vi "Begin.vi"(8 "error in":errorcluster) -> (0 "error out":errorcluster)   [LabVIEW 2016]
doc: "Called before other user functions, this VI is expected to open initial I/O refnums, load in file data, and do all program initialization. Notice that the <B>error out</B> terminal is simply used for data flow. Wiring it to other structures or subVIs ensures that this VI runs first."
uses:
  <vilib>/Rock Robotics/WPI/Joystick/WPI_JoystickDeviceEnum.ctl
  <vilib>/Rock Robotics/WPI/ThirdParty/Sensors/navX/_TypeDefs/FRIC_navX_DeviceNumbersTypeDef.ctl
  <vilib>/Rock Robotics/WPI/ThirdParty/CanMotor/TalonSRX/WPI_CANTalonSRX_APIControlMode.ctl
  <vilib>/Rock Robotics/WPI/ThirdParty/CanMotor/TalonSRX/WPI_CANTalonSRX_BrakeOverride.ctl
  <vilib>/Rock Robotics/SystemInterfaces/DIO/FPGA_DIOPWMChannel.ctl
  <vilib>/Rock Robotics/WPI/SafetyOutput/WPI_SafetyOutputConfigMenu.ctl
  <vilib>/Rock Robotics/WPI/DriverStation/WPI_DriverStationRobotMode2.ctl
  <vilib>/Rock Robotics/Network Tables/NT Write String Array.vi
  Robot Global Data.vi
  <vilib>/Rock Robotics/WPI/Camera/WPI_CameraFrameRate.ctl
  <vilib>/Rock Robotics/WPI/Camera/WPI_CameraImageSize.ctl
  <vilib>/Rock Robotics/WPI/Camera/WPI_CameraWhite Balance Values.ctl
  <vilib>/Rock Robotics/WPI/Camera/WPI_CameraExposure Values.ctl
  <vilib>/Rock Robotics/WPI/RobotDrive/WPI_RobotDriveOpen2MotorWithTalon.vi
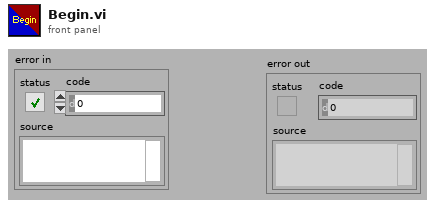
[diagram p1: front panel]
types:
  T1 = typedef "WPI_DriverStationRobotMode2.ctl" = enum16{"Autonomous Disabled", "Autonomous Enabled", "Teleop Disabled", "Teleop Enabled", "Disconnected", "Finish", "Test Disabled", "Test Enabled", "Emergency Stopped"}
  T2 = typedef "WPI_SafetyOutputConfigMenu.ctl" = enum16{"Enable", "Disable"}
  T3 = typedef "FPGA_DIOPWMChannel.ctl" = enum8{"PWM 0", "PWM 1", "PWM 2", "PWM 3", "PWM 4", "PWM 5", "PWM 6", "PWM 7", "PWM 8", "PWM 9", "PWM MXP 0", "PWM MXP 1", "PWM MXP 2", "PWM MXP 3", "PWM MXP 4", "PWM MXP 5", "PWM MXP 6", "PWM MXP 7", "PWM MXP 8", "PWM MXP 9", "Invalid"}
  T4 = typedef "WPI_RobotDriveDevRef.ctl" = cluster{"DevStatus":errorcluster, "Motors[]":T5[], "Square Inputs":bool, "Max Output":dbl}
  T5 = typedef "WPI_MotorControlDeviceRef.ctl" = cluster{"DeviceStatus":errorcluster, "Type":T6, "PWM":cluster{"PWM Channel":T3, "DeadBand":T7}, "CAN":cluster{"Device Number":u8, "SetOutput VI Ref":variant, "GetOutput VI Ref":variant, "Enable VI Ref":variant, "Disable VI Ref":variant, "Data":variant}, "Invert":bool}
  T6 = typedef "WPI_MotorControlType.ctl" = enum16{"PWM", "CAN"}
  T7 = typedef "WPI_PWMDeadband.ctl" = cluster{"Name":string, "maxPositivePwm":i32, "minPositivePwm":i32, "centerPwm":i32, "maxNegativePwm":i32, "minNegativePwm":i32, "angularRange":u16}
  T8 = typedef "WPI_CANTalonSRX_BrakeOverride.ctl" = enum8{"No Override", "Override to Coast", "Override to Brake"}
  T9 = typedef "WPI_CANTalonSRX_APIControlMode.ctl" = enum8{"Percent VBus", "Speed", "Position", "Slave", "Unchanged / Invalid", "Voltage Compensation", "Current", "Motion Profile", "Motion Magic"}
  T10 = typedef "WPI_CameraExposure Values.ctl" = enum16{"Auto", "Flicker-free 50 Hz", "Flicker-free 60 Hz", "Hold current", "Custom"}
  T11 = typedef "WPI_CameraWhite Balance Values.ctl" = enum16{"Auto", "Fixed indoor", "Fixed outdoor 1", "Fixed outdoor 2", "Fixed fluorescent 1", "Fixed fluorescent 2", "Hold current", "Custom"}
  T12 = typedef "WPI_CameraImageSize.ctl" = enum16{"640x480", "320x240", "160x120", "Custom"}
  T13 = typedef "WPI_CameraFrameRate.ctl" = u32
  T14 = typedef "WPI_CameraDevRef.ctl" = cluster{"Camera Address":string, "CameraStatus":errorcluster}
  T15 = typedef "WPI_JoystickDeviceEnum.ctl" = enum16{"USB 0", "USB 1", "USB 2", "USB 3", "USB 4", "USB 5"}
  T16 = typedef "WPI_JoystickDevRef.ctl" = cluster{"Device":T15}
  T17 = typedef "FRIC_navX_DeviceNumbersTypeDef.ctl" = enum16{"Dev0", "Dev1", "Dev2", "Dev3"}
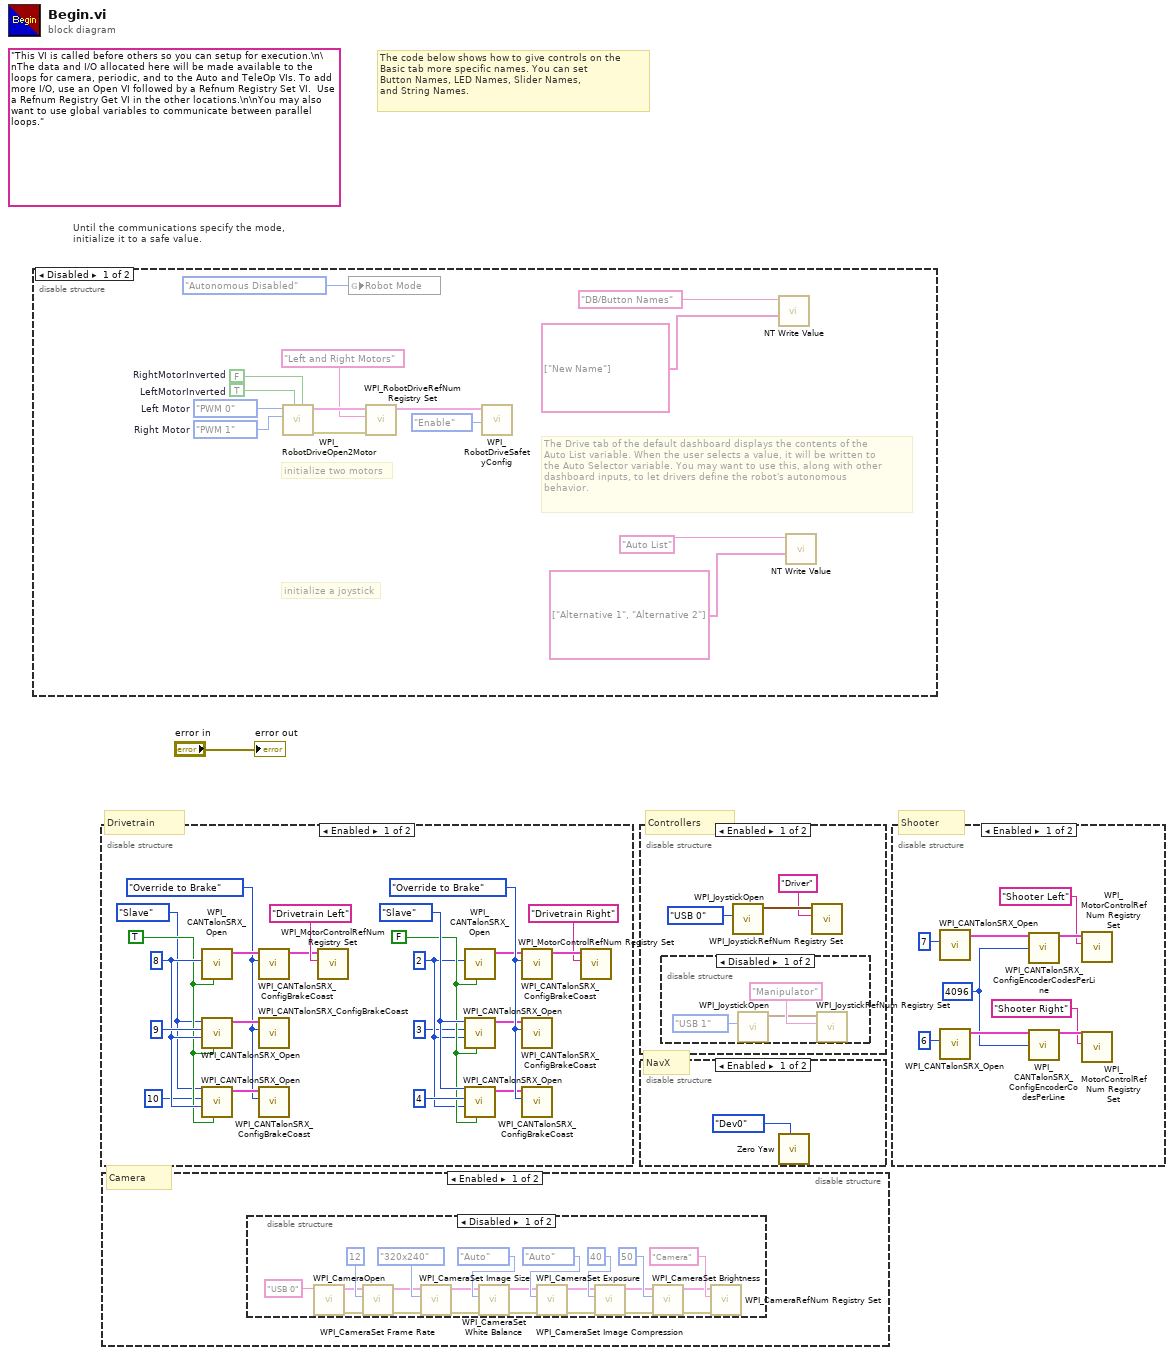
[diagram p0: block diagram]
diagram:
  (unwired) "This VI is called before others so you can setup for execution.\n\nThe data and I/O allocated here will be made available to the loops for camera, periodic, and to the Auto and TeleOp VIs. To add more I/O, use an Open VI followed by a Refnum Registry Set VI.  Use a Refnum Registry Get VI in the other locations.\n\nYou may also want to use global variables to communicate between parallel loops."
  # "NavX"
  # "Shooter"
  # "Camera"
  # "Drivetrain"
  # "Controllers"
  # "The code below shows how to give controls on the\nBasic tab more specific names. You can set\nButton Names, LED Names, Slider Names,\nand String Names."
  # "Until the communications specify the mode,\ninitialize it to a safe value."
  n1 = disable-structure shown="Disabled" {
    frame Disabled {
      w9 = FPGA_DIOPWMChannel."PWM 1"  # Right Motor
      w10 = FPGA_DIOPWMChannel."PWM 0"  # Left Motor
      w14 = TRUE  # LeftMotorInverted
      w15 = FALSE  # RightMotorInverted
      # "The Drive tab of the default dashboard displays the contents of the\nAuto List variable. When the user selects a value, it will be written to\nthe Auto Selector variable. You may want to use this, along with other\ndashboard inputs, to let drivers define the robot's autonomous\nbehavior."
      # "initialize a joystick"
      # "initialize two motors"
      n2 = call-poly <vilib>:"WPI_RobotDriveOpen2Motor.vi"("Right Motor Inverted"=w15, "Left Motor Inverted"=w14, "Right Motor"=w9, "Left Motor"=w10) -> ("error out"=w11:errorcluster, "RobotDriveDevRef"=w13:T4)  [unwired: 1 in, 5 out]
      n3 = global write "Robot Global Data.vi" "Robot Mode"(WPI_DriverStationRobotMode2."Autonomous Disabled" ("Robot Mode")) -> ()
      n4 = call <vilib>:"WPI_RobotDriveRefNum Registry Set.vi"("error in (no error)"=w11, "refnum name"="Left and Right Motors", "RobotDriveDevRef"=w13) -> ("RobotDriveDevRef"=w8:T4)  [unwired: 1 in, 7 out]
      n5 = call <vilib>:"WPI_RobotDriveSafetyConfig.vi"("mode"=WPI_SafetyOutputConfigMenu."Enable", "RobotDriveDevRef"=w8) -> ()  [unwired: 8 in, 2 out]
      n6 = call-poly <vilib>:"NT Write Value.vi"("String Array"=string[] ["New Name"], "Name"="DB/Button Names") -> ()  [unwired: 9 in, 1 out]
      n7 = call-poly <vilib>:"NT Write Value.vi"("String Array"=string[] ["Alternative 1", "Alternative 2"], "Name"="Auto List") -> ()  [unwired: 9 in, 1 out]
    }
    frame Enabled {
    }
  }
  n8 = disable-structure shown="Enabled" {
    frame Enabled {
      w26 = WPI_CANTalonSRX_BrakeOverride."Override to Brake" ("Brake / Coast Mode")
      w20 = FALSE ("Invert")
      w22 = WPI_CANTalonSRX_APIControlMode."Slave" ("Control Mode")
      w17 = u8 2 ("Device Number")
      w27 = WPI_CANTalonSRX_BrakeOverride."Override to Brake" ("Brake / Coast Mode")
      w33 = TRUE ("Invert")
      w31 = WPI_CANTalonSRX_APIControlMode."Slave" ("Control Mode")
      w36 = u8 8 ("Device Number")
      n9 = call <vilib>:"WPI_CANTalonSRX_Open.vi"("Invert"=w33, "Device Number"=w36) -> ("CAN Talon SRX Ref"=w35:T5)  [unwired: 8 in, 1 out]
      n10 = call <vilib>:"WPI_CANTalonSRX_Open.vi"("Invert"=w33, "Master Device Number"=w36, "Device Number"=u8 9, "Control Mode"=w31) -> ("CAN Talon SRX Ref"=w30:T5)  [unwired: 6 in, 1 out]
      n11 = call <vilib>:"WPI_CANTalonSRX_Open.vi"("Invert"=w33, "Master Device Number"=w36, "Device Number"=u8 10, "Control Mode"=w31) -> ("CAN Talon SRX Ref"=w28:T5)  [unwired: 6 in, 1 out]
      n12 = call <vilib>:"WPI_CANTalonSRX_ConfigBrakeCoast.vi"("Brake / Coast Mode"=w27, "CAN Talon SRX Ref"=w35) -> ("CAN Talon SRX Ref"=w29:T5)  [unwired: 8 in, 1 out]
      n13 = call <vilib>:"WPI_CANTalonSRX_ConfigBrakeCoast.vi"("Brake / Coast Mode"=w27, "CAN Talon SRX Ref"=w30) -> ()  [unwired: 8 in, 2 out]
      n14 = call <vilib>:"WPI_CANTalonSRX_ConfigBrakeCoast.vi"("Brake / Coast Mode"=w27, "CAN Talon SRX Ref"=w28) -> ()  [unwired: 8 in, 2 out]
      n15 = call <vilib>:"WPI_MotorControlRefNum Registry Set.vi"("refnum name"="Drivetrain Left", "MotorControlDevRef"=w29) -> ()  [unwired: 8 in, 2 out]
      n16 = call <vilib>:"WPI_CANTalonSRX_Open.vi"("Invert"=w20, "Device Number"=w17) -> ("CAN Talon SRX Ref"=w18:T5)  [unwired: 8 in, 1 out]
      n17 = call <vilib>:"WPI_CANTalonSRX_Open.vi"("Invert"=w20, "Master Device Number"=w17, "Device Number"=u8 3, "Control Mode"=w22) -> ("CAN Talon SRX Ref"=w23:T5)  [unwired: 6 in, 1 out]
      n18 = call <vilib>:"WPI_CANTalonSRX_Open.vi"("Invert"=w20, "Master Device Number"=w17, "Device Number"=u8 4, "Control Mode"=w22) -> ("CAN Talon SRX Ref"=w25:T5)  [unwired: 6 in, 1 out]
      n19 = call <vilib>:"WPI_CANTalonSRX_ConfigBrakeCoast.vi"("Brake / Coast Mode"=w26, "CAN Talon SRX Ref"=w18) -> ("CAN Talon SRX Ref"=w24:T5)  [unwired: 8 in, 1 out]
      n20 = call <vilib>:"WPI_CANTalonSRX_ConfigBrakeCoast.vi"("Brake / Coast Mode"=w26, "CAN Talon SRX Ref"=w23) -> ()  [unwired: 8 in, 2 out]
      n21 = call <vilib>:"WPI_CANTalonSRX_ConfigBrakeCoast.vi"("Brake / Coast Mode"=w26, "CAN Talon SRX Ref"=w25) -> ()  [unwired: 8 in, 2 out]
      n22 = call <vilib>:"WPI_MotorControlRefNum Registry Set.vi"("refnum name"="Drivetrain Right", "MotorControlDevRef"=w24) -> ()  [unwired: 8 in, 2 out]
    }
    frame Disabled {
    }
  }
  n23 = disable-structure shown="Enabled" {
    frame Enabled {
      n24 = disable-structure shown="Disabled" {
        frame Disabled {
          n25 = call <vilib>:"WPI_CameraOpen.vi"("Camera Address"="USB 0") -> ("error out"=w50:errorcluster, "CameraDevRef"=w51:T14)  [unwired: 9 in]
          n26 = call <vilib>:"WPI_CameraSet Frame Rate.vi"("error in (no error)"=w50, "Frame Rate (fps)"=T13 12, "CameraDevRef"=w51) -> ("error out"=w48:errorcluster, "CameraDevRef Out"=w49:T14)  [unwired: 7 in]
          n27 = call <vilib>:"WPI_CameraSet Image Size.vi"("error in (no error)"=w48, "Image Size"=WPI_CameraImageSize."320x240", "CameraDevRef"=w49) -> ("error out"=w46:errorcluster, "CameraDevRef Out"=w47:T14)  [unwired: 7 in]
          n28 = call <vilib>:"WPI_CameraSet White Balance.vi"("error in (no error)"=w46, "White Balance"=WPI_CameraWhite_Balance_Values."Auto", "CameraDevRef"=w47) -> ("error out"=w44:errorcluster, "CameraDevRef Out"=w45:T14)  [unwired: 7 in]
          n29 = call <vilib>:"WPI_CameraSet Exposure.vi"("error in (no error)"=w44, "Exposure"=WPI_CameraExposure_Values."Auto", "CameraDevRef"=w45) -> ("error out"=w42:errorcluster, "CameraDevRef Out"=w43:T14)  [unwired: 7 in]
          n30 = call <vilib>:"WPI_CameraSet Image Compression.vi"("error in (no error)"=w42, "Compression"=40, "CameraDevRef"=w43) -> ("error out"=w40:errorcluster, "CameraDevRef Out"=w41:T14)  [unwired: 7 in]
          n31 = call <vilib>:"WPI_CameraSet Brightness.vi"("error in (no error)"=w40, "Brightness"=50, "CameraDevRef"=w41) -> ("error out"=w38:errorcluster, "CameraDevRef Out"=w39:T14)  [unwired: 7 in]
          n32 = call <vilib>:"WPI_CameraRefNum Registry Set.vi"("error in (no error)"=w38, "refnum name"="Camera", "CameraDevRef"=w39) -> ()  [unwired: 7 in, 2 out]
        }
        frame Enabled {
        }
      }
    }
    frame Disabled {
    }
  }
  n33 = disable-structure shown="Enabled" {
    frame Enabled {
      n34 = disable-structure shown="Disabled" {
        frame Disabled {
          n35 = call <vilib>:"WPI_JoystickOpen.vi"("JoystickDevice"=WPI_JoystickDeviceEnum."USB 1") -> ("JoystickDevRef"=w64:T16)  [unwired: 10 in]
          n36 = call <vilib>:"WPI_JoystickRefNum Registry Set.vi"("refnum name"="Manipulator", "JoystickDevRef"=w64) -> ()  [unwired: 8 in, 2 out]
        }
        frame Enabled {
        }
      }
      n37 = call <vilib>:"WPI_JoystickOpen.vi"("JoystickDevice"=WPI_JoystickDeviceEnum."USB 0") -> ("JoystickDevRef"=w61:T16)  [unwired: 10 in]
      n38 = call <vilib>:"WPI_JoystickRefNum Registry Set.vi"("refnum name"="Driver", "JoystickDevRef"=w61) -> ()  [unwired: 8 in, 2 out]
    }
    frame Disabled {
    }
  }
  n39 = disable-structure shown="Enabled" {
    frame Enabled {
      n40 = call <vilib>:"Zero Yaw.vi"("Device Number"=FRIC_navX_DeviceNumbersTypeDef."Dev0") -> ()  [unwired: 11 in]
    }
    frame Disabled {
    }
  }
  n41 = disable-structure shown="Enabled" {
    frame Enabled {
      w71 = 4096
      n42 = call <vilib>:"WPI_CANTalonSRX_Open.vi"("Device Number"=u8 7) -> ("CAN Talon SRX Ref"=w72:T5)  [unwired: 9 in, 1 out]
      n43 = call <vilib>:"WPI_CANTalonSRX_Open.vi"("Device Number"=u8 6) -> ("CAN Talon SRX Ref"=w75:T5)  [unwired: 9 in, 1 out]
      n44 = call <vilib>:"WPI_CANTalonSRX_ConfigEncoderCodesPerLine.vi"("CAN Talon SRX Ref"=w72, "Number Encoder Lines\n(Counts Per Rotation)"=w71) -> ("CAN Talon SRX Ref"=w73:T5)  [unwired: 12 in, 1 out]
      n45 = call <vilib>:"WPI_CANTalonSRX_ConfigEncoderCodesPerLine.vi"("CAN Talon SRX Ref"=w75, "Number Encoder Lines\n(Counts Per Rotation)"=w71) -> ("CAN Talon SRX Ref"=w74:T5)  [unwired: 12 in, 1 out]
      n46 = call <vilib>:"WPI_MotorControlRefNum Registry Set.vi"("refnum name"="Shooter Left", "MotorControlDevRef"=w73) -> ()  [unwired: 8 in, 2 out]
      n47 = call <vilib>:"WPI_MotorControlRefNum Registry Set.vi"("refnum name"="Shooter Right", "MotorControlDevRef"=w74) -> ()  [unwired: 8 in, 2 out]
    }
    frame Disabled {
    }
  }
  "error out" <- "error in"
